vi "find next action.vi"(10 "desired state":T1, 11 "current state":T1) -> (3 "action":T2)   [LabVIEW 2013, in "main engine.lvlib"]
uses:
  main engine/main engine.lvlib
  engine process action.ctl
  engine state.ctl
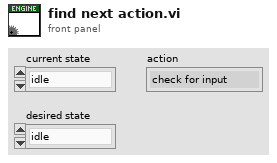
[diagram p1: front panel]
types:
  T1 = typedef "main engine.lvlib/engine state.ctl" = enum16{"idle", "configured", "running", "safe state", "exit"}
  T2 = typedef "main engine.lvlib/engine process action.ctl" = enum16{"check for input", "load configuration", "unload configuration", "set safe outputs", "pre-run", "timed loop", "quit"}
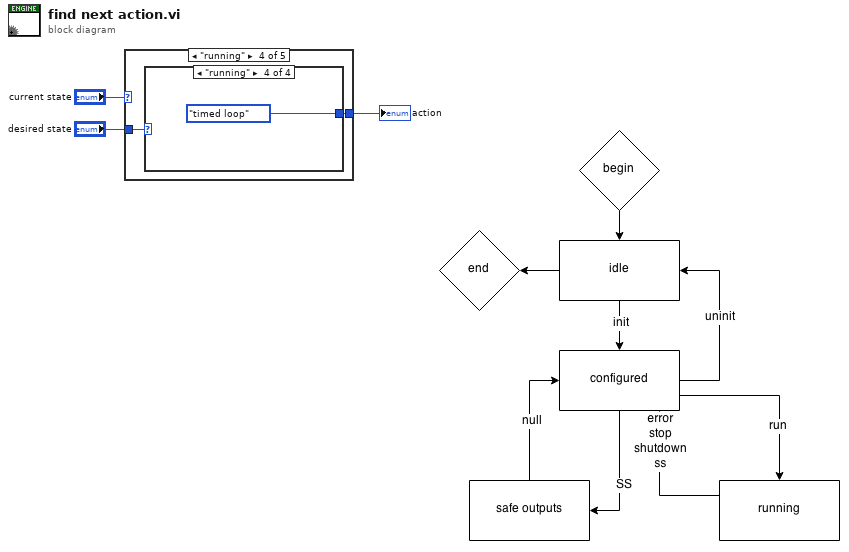
[diagram p0: block diagram]
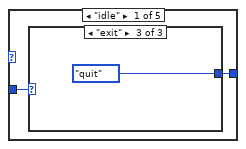
[diagram p2: hidden frame]
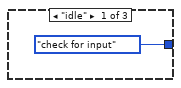
[diagram p3: hidden frame]
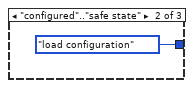
[diagram p4: hidden frame]
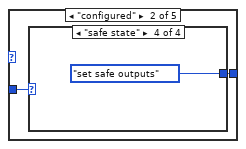
[diagram p5: hidden frame]
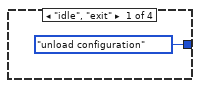
[diagram p6: hidden frame]
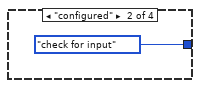
[diagram p7: hidden frame]
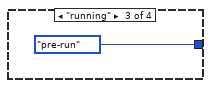
[diagram p8: hidden frame]
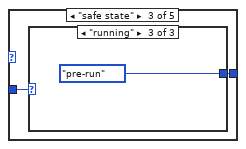
[diagram p9: hidden frame]
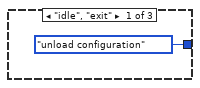
[diagram p10: hidden frame]
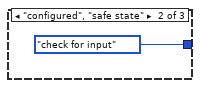
[diagram p11: hidden frame]
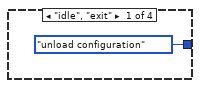
[diagram p12: hidden frame]
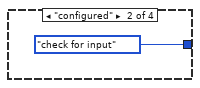
[diagram p13: hidden frame]
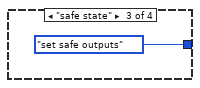
[diagram p14: hidden frame]
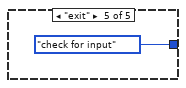
[diagram p15: hidden frame]
diagram:
  n1 = case shown="\"running\"" "current state" {
    tunnel: "desired state" -> [w5 w10 w16 w21 _]
    tunnel: [w4 w9 w15 w20 engine_process_action."check for input"] -> w1
    frame "idle" {
      n2 = case shown="\"exit\"" w5 {
        tunnel: [engine_process_action."check for input" engine_process_action."load configuration" engine_process_action."quit"] -> w4
        frame "idle" {
        }
        frame "configured".."safe state" {
        }
        frame "exit" {
        }
      }
    }
    frame "configured" {
      n3 = case shown="\"safe state\"" w10 {
        tunnel: [engine_process_action."unload configuration" engine_process_action."check for input" engine_process_action."pre-run" engine_process_action."set safe outputs"] -> w9
        frame "idle", "exit" {
        }
        frame "configured" {
        }
        frame "running" {
        }
        frame "safe state" {
        }
      }
    }
    frame "safe state" {
      n4 = case shown="\"running\"" w16 {
        tunnel: [engine_process_action."unload configuration" engine_process_action."check for input" engine_process_action."pre-run"] -> w15
        frame "idle", "exit" {
        }
        frame "configured", "safe state" {
        }
        frame "running" {
        }
      }
    }
    frame "running" {
      n5 = case shown="\"running\"" w21 {
        tunnel: [engine_process_action."unload configuration" engine_process_action."check for input" engine_process_action."set safe outputs" engine_process_action."timed loop"] -> w20
        frame "idle", "exit" {
        }
        frame "configured" {
        }
        frame "safe state" {
        }
        frame "running" {
        }
      }
    }
    frame "exit" {
    }
  }
  "action" <- w1
